vi "Configure Sweep Coupling.vi"(4 "Manual Video BW (1 MHz)":i32=1000000 format="%.0g", 5 "Manual Resolution BW (3 MHz)":i32=3000000 format="%.0g", 6 "Auto Video BW (T: Enable)":bool=TRUE, 7 "Auto Resolution BW (T: Enable)":bool=TRUE, 8 "error in (no error)":errorcluster, 9 "Manual Sweep Time (4 ms)":dbl=0.004, 10 "Auto Sweep Time (T: Enable)":bool=TRUE, 11 "VISA resource name":refnum<visa-resource-name>) -> (0 "error out":errorcluster, 3 "VISA resource name out":refnum<visa-resource-name>)   [LabVIEW 2013, in "Template - Spectrum Analyzer.lvlib"]
doc: "Configures the coupling and sweeping properties of the spectrum analyzer. Resolution bandwidth, video bandwidth, and sweep time can be coupled together by the instrument or set manually."
uses:
  <instrlib>/_Template - Spectrum Analyzer/Template - Spectrum Analyzer.lvlib
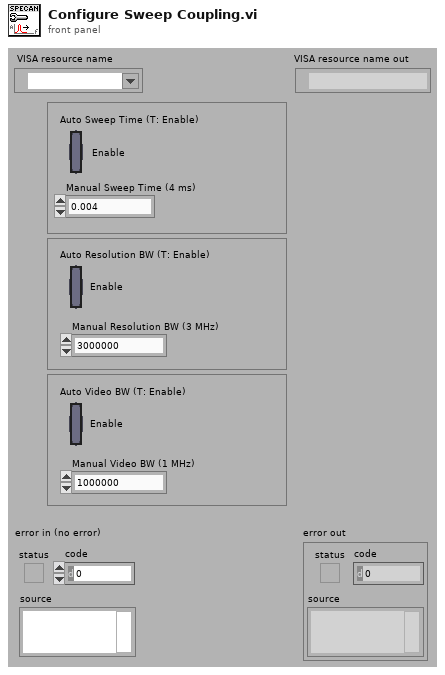
[diagram p1: front panel]
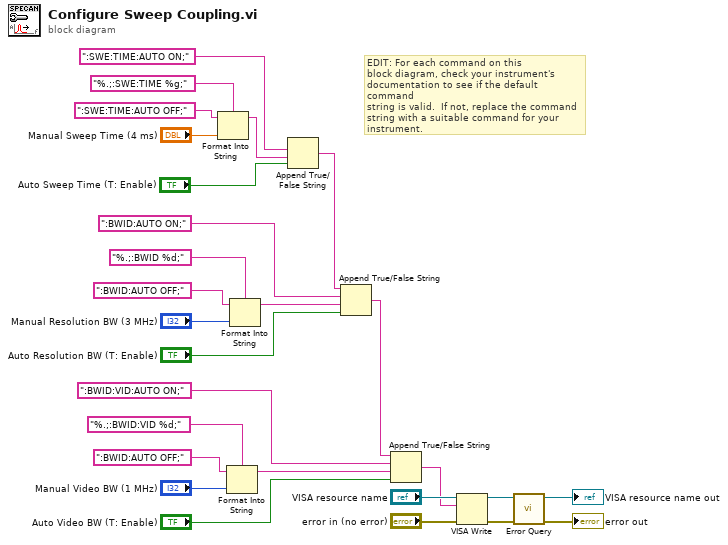
[diagram p0: block diagram]
diagram:
  # "EDIT: For each command on this\nblock diagram, check your instrument's\ndocumentation to see if the default command\nstring is valid.  If not, replace the command\nstring with a suitable command for your\ninstrument."
  n1 = Format Into String(format string="%.;:SWE:TIME %g;", initial string=":SWE:TIME:AUTO OFF;", "Manual Sweep Time (4 ms)") -> (resulting string=w4:string)  [unwired: 1 in, 1 out]
  n2 = Format Into String(format string="%.;:BWID:VID %d;", initial string=":BWID:AUTO OFF;" ("format string"), "Manual Video BW (1 MHz)") -> (resulting string=w20:string)  [unwired: 1 in, 1 out]
  n3 = Format Into String(format string="%.;:BWID %d;", initial string=":BWID:AUTO OFF;" ("format string"), "Manual Resolution BW (3 MHz)") -> (resulting string=w13:string)  [unwired: 1 in, 1 out]
  n4 = Append True/False String(1:"Auto Sweep Time (T: Enable)", 2:w4, 3:":SWE:TIME:AUTO ON;") -> (0:w1:string)  [unwired: 1 in]
  n5 = Append True/False String(1:"Auto Resolution BW (T: Enable)", 2:w13, 3:":BWID:AUTO ON;" ("format string"), 4:w1) -> (0:w12:string)
  n6 = Append True/False String(1:"Auto Video BW (T: Enable)", 2:w20, 3:":BWID:VID:AUTO ON;" ("format string"), 4:w12) -> (0:w19:string)
  n7 = VISA Write(VISA resource name="VISA resource name", write buffer=w19, error in (no error)="error in (no error)") -> (VISA resource name out=w9:refnum<visa-resource-name>, error out=w7:errorcluster)  [unwired: 1 out]
  n8 = call <instrlib>:"Error Query.vi"("error in (no error)"=w7, "VISA resource name"=w9) -> ("error out"=→"error out":errorcluster, "VISA resource name out"=→"VISA resource name out":refnum<visa-resource-name>)  [unwired: 6 in, 2 out]
